vi "JVParameters.vi"(1 "InputJV":dbl[][](array[numeric])) -> (0 "JVParameters":dbl[](array[numeric]))   [LabVIEW 2020]
uses:
  <vilib>/gmath/NI_Gmath.lvlib
panel:
  out "FF":sgl
  out "JMPP (mA/cm2)":sgl
  out "J_SC (mA/cm2)":sgl
  out "V_OC (V)":sgl
  out "PMax (mW/cm2)":sgl
  out "VMPP (V)":sgl
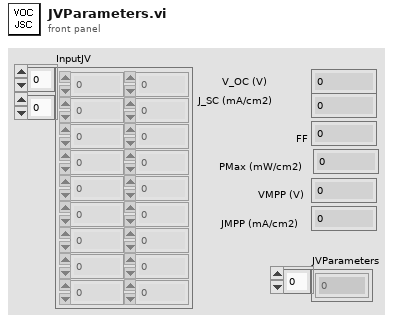
[diagram p1: front panel]
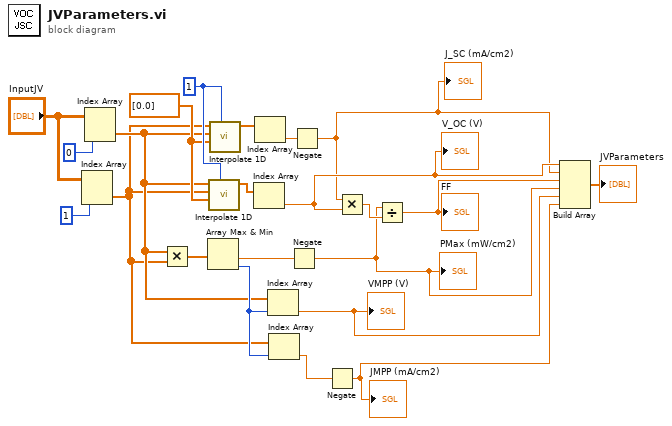
[diagram p0: block diagram]
diagram:
  w18 = dbl[] [0.0] ("xi")
  w19 = 1 ("disabled index (col)")
  n1 = Index Array(array="InputJV", index (col)=1 ("disabled index (col)")) -> (element=w14:dbl[])  [unwired: 1 in]
  n2 = Index Array(array="InputJV", index (col)=0 ("disabled index (col)")) -> (element=w15:dbl[])  [unwired: 1 in]
  n3 = Multiply(x=w15, y=w14) -> (x*y=w17:dbl[])
  n4 = Array Max & Min(array=w17) -> (min value=w13:dbl, min index (indices)=w16:i32)  [unwired: 2 out]
  n5 = call <vilib>:"Interpolate 1D.vi"("method"=w19, "xi"=w18, "X"=w14, "Y"=w15) -> ("yi"=w1:dbl[])  [unwired: 5 in, 2 out]
  n6 = call <vilib>:"Interpolate 1D.vi"("method"=w19, "xi"=w18, "X"=w15, "Y"=w14) -> ("yi"=w12:dbl[])  [unwired: 5 in, 2 out]
  n7 = Index Array(array=w1) -> (element=w9:dbl)  [unwired: 1 in]
  "V_OC (V)" <- w9
  n8 = Index Array(array=w12) -> (element=w11:dbl)  [unwired: 1 in]
  n9 = Index Array(array=w15, index=w16) -> (element=w5:dbl)
  "VMPP (V)" <- w5
  n10 = Index Array(array=w14, index=w16) -> (element=w4:dbl)
  n11 = Negate(x=w13) -> (-x=w6:dbl)
  "PMax (mW/cm2)" <- w6
  n12 = Negate(x=w11) -> (-x=w8:dbl)
  "J_SC (mA/cm2)" <- w8
  n13 = Negate(x=w4) -> (-x=w3:dbl)
  "JMPP (mA/cm2)" <- w3
  n14 = Multiply(x=w8, y=w9) -> (x*y=w10:dbl)
  n15 = Divide(x=w6, y=w10) -> (x/y=w7:dbl)
  "FF" <- w7
  n16 = Build Array(w9, w8, w7, w6, w5, w3) -> (→"JVParameters":dbl[])
